vi "CMD StopLog.vi"(8 "error in (no error)":errorcluster, 10 "bypass (F)":bool, 11 "Log_Engine in":refnum<class "Log_Engine.lvclass">) -> (0 "error out":errorcluster, 3 "Log_Engine out":refnum<class "Log_Engine.lvclass">)   [LabVIEW 2019, in "Log_Engine.lvclass"]
doc: "Developed by Kevin Thompson\nkevin@thompsonengineering.net\n\nCopyright 2018\nThompson Engineering, LLC"
uses:
  Log_Engine.lvclass
  DataTypes/AsynCmd_Log_Engine--enum.ctl
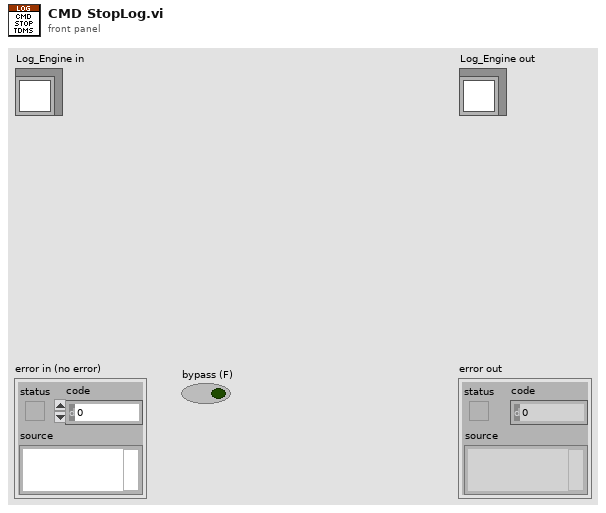
[diagram p1: front panel]
types:
  T1 = typedef "Log_Engine.lvclass/AsynCmd_Log_Engine--enum.ctl" = enum16{"Log_Engine.StartLog", "Log_Engine.StopLog", "Log_Engine.StartESRLog", "Log_Engine.StopESRLog"}
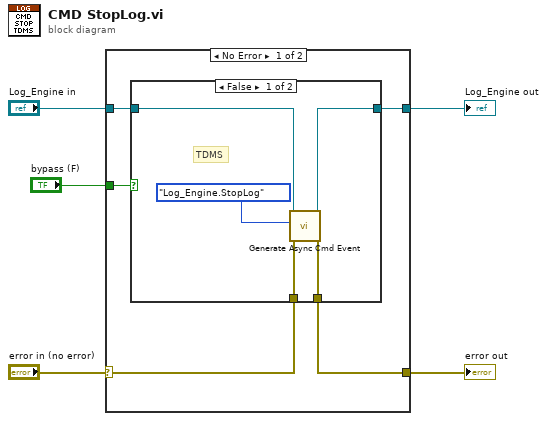
[diagram p0: block diagram]
diagram:
  n1 = case shown="No Error" "error in (no error)" {
    selector: "error in (no error)" -> [w8 w19]
    tunnel: [w7 w19] -> w4
    tunnel: [w9 w18] -> w2
    tunnel: "Log_Engine in" -> [w10 w18]
    tunnel: "bypass (F)" -> [w6 _]
    frame No Error {
      n2 = case shown="False" w6 {
        tunnel: w10 -> [w15 w16]
        tunnel: [w14 w16] -> w9
        tunnel: w8 -> [w13 w17]
        tunnel: [w12 w17] -> w7
        frame False {
          # "TDMS"
          n3 = call "Generate Async Cmd Event.vi"("error in (no error)"=w13, "AsyncCmd"=AsynCmd_Log_Engine--enum."Log_Engine.StopLog", "Log_Engine in"=w15) -> ("error out"=w12:errorcluster, "Log_Engine out"=w14:refnum<class "Log_Engine.lvclass">)  [unwired: 7 in]
        }
        frame True {
        }
      }
    }
    frame Error {
    }
  }
  "error out" <- w4
  "Log_Engine out" <- w2
